vi "Send Toggle Output.vi"(8 "error in":errorcluster, 11 "69X_79X in":refnum<class "79XRP.lvclass">) -> (0 "error out":errorcluster, 3 "69X_79X out":refnum<class "79XRP.lvclass">)   [LabVIEW 2019, in "79XRP.lvlib" / "79XRP.lvclass"]
uses:
  Library/79XRP.lvclass
  C:/Users/Public/Documents/Development/builds/Instruments/PowerSupply.lvlibp/Library/PowerSupply.lvclass
  Accessors/Read Local Resource.vi
  Accessors/Write Local Resource.vi
  <instrlib>/Keysight RP7900 Series/Keysight RP7900 Series.lvlib
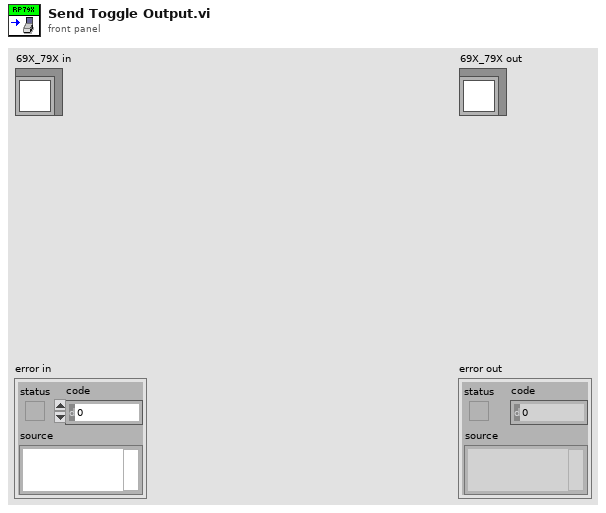
[diagram p1: front panel]
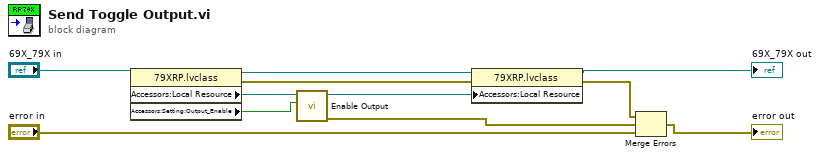
[diagram p0: block diagram]
diagram:
  n1 = property class="79XRP.lvclass"(reference="69X_79X in") -> (reference out=w10:refnum<class "79XRP.lvclass">, error out=w9:errorcluster, "Accessors:Local Resource"=w1:refnum<visa-resource-name>, "Accessors:Setting:Output_Enable"=w2:bool)  [unwired: 1 in]
  n2 = call <instrlib>:"Enable Output.vi"("Enable Output (F: Disable)"=w2, "VISA resource name"=w1) -> ("error out"=w4:errorcluster, "VISA resource name out"=w5:refnum<visa-resource-name>)  [unwired: 8 in]
  n3 = property class="79XRP.lvclass"(reference=w10, error in=w9, "Accessors:Local Resource"=w5) -> (reference out=→"69X_79X out":refnum<class "79XRP.lvclass">, error out=w7:errorcluster)
  n4 = Merge Errors(w7, w4, "error in") -> (→"error out":errorcluster)
